vi "Is String Data Source Terminal Connected to Add States SubVI.vi"(7 "Wires Traversed in (for recursion)":refnum<vi>[](array[refnum]), 8 "error in (no error)":errorcluster, 11 "Wire":refnum<vi>) -> (0 "error out":errorcluster, 2 "Connected to Add States?":bool, 3 "Add States SubVI":refnum<vi>, 5 "Wires Traversed out":refnum<vi>[](array[refnum]))   [LabVIEW 2013, in "JKI State Machine API.lvlib"]
uses:
  JKI State Machine API.lvlib
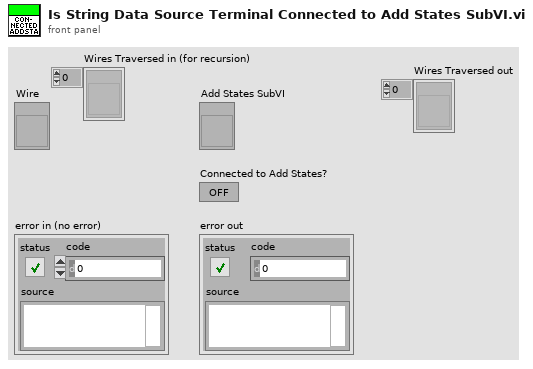
[diagram p1: front panel]
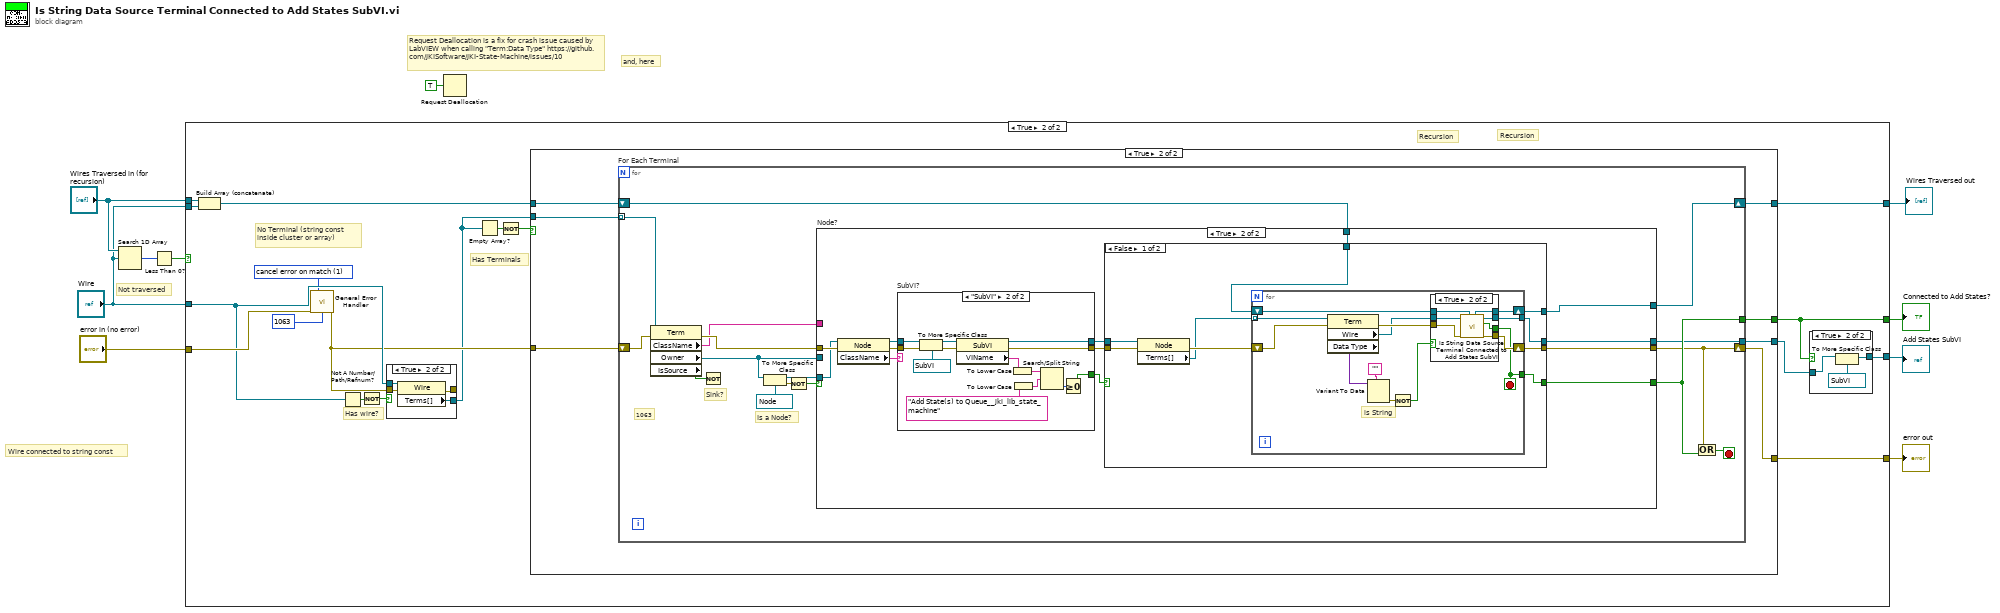
[diagram p0: block diagram]
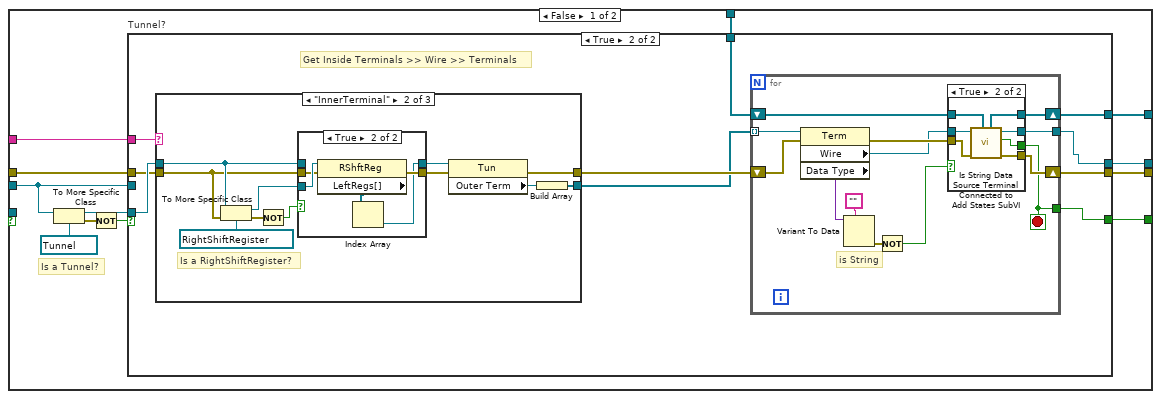
[diagram p5: hidden frame]
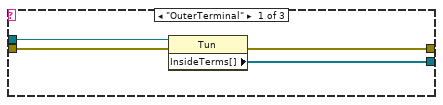
[diagram p7: hidden frame]
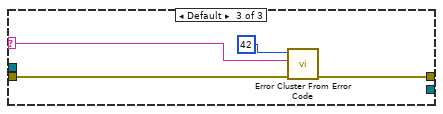
[diagram p9: hidden frame]
diagram:
  # "and, here"
  # "Request Deallocation is a fix for crash issue caused by LabVIEW when calling \"Term:Data Type\" https://github.com/JKISoftware/JKI-State-Machine/issues/10"
  # "Not traversed"
  # "Wire connected to string const"
  n1 = Search 1D Array(1D array="Wires Traversed in (for recursion)", element="Wire") -> (index of element=w6:i32)  [unwired: 1 in]
  n2 = Less Than 0?(x=w6) -> (x < 0?=w5:bool)
  n3 = case shown="True" w5 {
    tunnel: "error in (no error)" -> [w11 w30]
    tunnel: "Wire" -> [_ w29]
    tunnel: [w11 w21] -> w9
    tunnel: [_ w20] -> w8
    tunnel: [_ w18] -> w7
    tunnel: "Wires Traversed in (for recursion)" -> [w12 w16]
    tunnel: "Wire" -> [_ w15]
    tunnel: [w12 w13] -> w2
    frame False {
    }
    frame True {
      w22 = 1 items=["no exception", "cancel error on match", "set error on match"] ("[exception action] (none:0)")
      # "Recursion"
      # "Recursion"
      # "Has Terminals"
      # "Has wire?"
      # "No Terminal (string const inside cluster or array)"
      n4 = Build Array (concatenate)(w16, w15) -> (w14:refnum<vi>[])
      n5 = call <vilib>:"General Error Handler.vi"("error in (no error)"=w30, "[exception action] (none:0)"=w22, "[exception code]"=1063 ("[error code] (0)")) -> ("error out"=w23:errorcluster)  [unwired: 8 in, 4 out]
      n6 = Not A Number/Path/Refnum?(number/path/refnum=w29) -> (NaN/Path/Refnum?=w25:bool)
      n7 = Not(x=w25) -> (.not. x?=w26:bool)
      n8 = case shown="True" w26 {
        tunnel: w29 -> [_ w197]
        tunnel: [_ w196] -> w17
        tunnel: [w193 w194] -> _
        tunnel: w23 -> [w193 w195]
        frame False {
        }
        frame True {
          n9 = property class="Wire"(reference=w197, error in=w195) -> (error out=w194:errorcluster, "Terms[]"=w196:refnum<vi>[])  [unwired: 1 out]
        }
      }
      n10 = Empty Array?(array=w17) -> (empty?=w27:bool)
      n11 = Not(x=w27) -> (.not. x?=w28:bool)
      n12 = case shown="True" w28 {
        tunnel: [_ w41] -> w20
        tunnel: [_ w40] -> w21
        tunnel: w23 -> [_ w39]
        tunnel: w17 -> [_ w37]
        tunnel: [_ w38] -> w19
        tunnel: w14 -> [w34 w36]
        tunnel: [w34 w35] -> w13
        frame False {
        }
        frame True {
          n13 = for "For Each Terminal" {
            shift-right: [w52] -> w40
            shift-left: w39 -> [w56]
            tunnel: [w53] -> w41
            tunnel: [w51] -> w38
            tunnel: w37 -> [w50] mode=indexing
            shift-right: [w42] -> w35
            shift-left: w36 -> [w43]
            stop <- w49 stop-if-true
            # "Is a Node?"
            # "1063"
            # "Sink?"
            n14 = property class="Term"(reference=w50, error in=w56) -> (error out=w57:errorcluster, "ClassName"=w48:string, "Owner"=w55:refnum<vi>, "IsSource"=w54:bool)  [unwired: 1 out]
            n15 = Not(x=w54) -> ()  [unwired: 1 out]
            n16 = To More Specific Class(target class=refnum<vi> refnum ("Node Refnum"), reference=w55) -> (specific class reference=w44:refnum<vi>, error out=w46:errorcluster)  [unwired: 1 in]
            n17 = Not(x=w46) -> (.not. x?=w45:bool)
            n18 = case "Node?" shown="True" w45 {
              tunnel: w57 -> [w64 w139]
              tunnel: [w63 w137] -> w52
              tunnel: [w61 w134] -> w53
              tunnel: w44 -> [_ w138]
              tunnel: w55 -> [w66 _]
              tunnel: [w62 w133] -> w51
              tunnel: w48 -> [w60 _]
              tunnel: w43 -> [w59 w131]
              tunnel: [w58 w130] -> w42
              frame False {
                # "Is a Tunnel?"
                n19 = To More Specific Class(target class=refnum<vi> refnum ("Tun Refnum"), reference=w66) -> (specific class reference=w67:refnum<vi>, error out=w69:errorcluster)  [unwired: 1 in]
                n20 = Not(x=w69) -> (.not. x?=w65:bool)
                n21 = case "Tunnel?" shown="True" w65 {
                  tunnel: w67 -> [_ w81]
                  tunnel: w66 -> [_ _]
                  tunnel: w64 -> [w71 w80]
                  tunnel: [w71 w78] -> w63
                  tunnel: [_ w77] -> w62
                  tunnel: [_ w76] -> w61
                  tunnel: w60 -> [_ w75]
                  tunnel: w59 -> [w70 w73]
                  tunnel: [w70 w72] -> w58
                  frame False {
                  }
                  frame True {
                    # "Get Inside Terminals >> Wire >> Terminals"
                    n22 = case shown="\"InnerTerminal\"" w75 {
                      selector: w75 -> [_ _ w105]
                      tunnel: w81 -> [w85 w93 _]
                      tunnel: w80 -> [w84 w91 w107]
                      tunnel: [w83 w96 w106] -> w79
                      tunnel: [w82 w94 _] -> w74
                      frame "OuterTerminal" {
                        n23 = property class="Tun"(reference=w85, error in=w84) -> (error out=w83:errorcluster, "InsideTerms[]"=w82:refnum<vi>[])  [unwired: 1 out]
                      }
                      frame "InnerTerminal" {
                        # "Is a RightShiftRegister?"
                        n24 = To More Specific Class(target class=refnum<vi> refnum ("RShftReg Refnum"), reference=w93, error in=w91) -> (specific class reference=w86:refnum<vi>, error out=w89:errorcluster)
                        n25 = Not(x=w89) -> (.not. x?=w87:bool)
                        n26 = case shown="True" w87 {
                          tunnel: w86 -> [_ w103]
                          tunnel: w93 -> [w98 _]
                          tunnel: [w98 w99] -> w92
                          tunnel: w91 -> [w97 w101]
                          tunnel: [w97 w100] -> w90
                          frame False {
                          }
                          frame True {
                            n27 = property class="RShftReg"(reference=w103, error in=w101) -> (error out=w100:errorcluster, "LeftRegs[]"=w102:refnum<vi>[])  [unwired: 1 out]
                            n28 = Index Array(array=w102) -> (element=w99:refnum<vi>)  [unwired: 1 in]
                          }
                        }
                        n29 = property class="Tun"(reference=w92, error in=w90) -> (error out=w96:errorcluster, "Outer Term"=w95:refnum<vi>)  [unwired: 1 out]
                        n30 = Build Array(w95) -> (w94:refnum<vi>[])
                      }
                      frame Default {
                        n31 = call <vilib>:"Error Cluster From Error Code.vi"("error in (no error)"=w107, "error message (\"\")"=w105, "error code (0)"=42) -> ("error out"=w106:errorcluster)  [unwired: 6 in]
                      }
                    }
                    n32 = for {
                      tunnel: w74 -> [w120] mode=indexing
                      shift-right: [w117] -> w78
                      shift-left: w79 -> [w119]
                      tunnel: [w116] -> w77
                      tunnel: [w115] -> w76
                      shift-right: [w112] -> w72
                      shift-left: w73 -> [w113]
                      stop <- w115 stop-if-true
                      # "is String"
                      n33 = property class="Term"(reference=w120, error in=w119) -> (error out=w118:errorcluster, "Wire"=w114:refnum<vi>, "Data Type"=w109:variant)  [unwired: 1 out]
                      n34 = Variant To Data(type="" ("error in (no error)"), Variant=w109) -> (error out=w110:errorcluster)  [unwired: 1 in, 1 out]
                      n35 = Not(x=w110) -> (.not. x?=w108:bool)
                      n36 = case shown="True" w108 {
                        tunnel: w114 -> [_ w125]
                        tunnel: w118 -> [w122 w129]
                        tunnel: [w122 w128] -> w117
                        tunnel: [_ w127] -> w115
                        tunnel: [_ w126] -> w116
                        tunnel: w113 -> [w121 w124]
                        tunnel: [w121 w123] -> w112
                        frame False {
                        }
                        frame True {
                          n37 = call "Is String Data Source Terminal Connected to Add States SubVI.vi"("Wires Traversed in (for recursion)"=w124, "error in (no error)"=w129, "Wire"=w125) -> ("error out"=w128:errorcluster, "Connected to Add States?"=w127:bool, "Add States SubVI"=w126:refnum<vi>, "Wires Traversed out"=w123:refnum<vi>[])  [unwired: 5 in]
                        }
                      }
                    }
                  }
                }
              }
              frame True {
                n38 = property class="Node"(reference=w138, error in=w139) -> (reference out=w141:refnum<vi>, error out=w140:errorcluster, "ClassName"=w142:string)
                n39 = case "SubVI?" shown="\"SubVI\"" w142 {
                  tunnel: w141 -> [w178 w191]
                  tunnel: w140 -> [w179 w188]
                  tunnel: [_ w180] -> w135
                  tunnel: [w179 w185] -> w136
                  tunnel: [w178 w184] -> w132
                  frame Default {
                  }
                  frame "SubVI" {
                    n40 = To More Specific Class(target class=refnum<vi> refnum ("SubVI Refnum"), reference=w191, error in=w188) -> (specific class reference=w190:refnum<vi>, error out=w189:errorcluster)
                    n41 = property class="SubVI"(reference=w190, error in=w189) -> (reference out=w184:refnum<vi>, error out=w185:errorcluster, "VIName"=w187:string)
                    n42 = To Lower Case(string=w187) -> (all lower case string=w183:string)
                    n43 = To Lower Case(string="Add State(s) to Queue__jki_lib_state_machine" ("VI Name")) -> (all lower case string=w182:string)
                    n44 = Search/Split String(string=w183, search string/char (-)=w182) -> (offset of match=w181:i32)  [unwired: 1 in, 2 out]
                    n45 = Greater Or Equal To 0?(x=w181) -> (x >= 0?=w180:bool)
                  }
                }
                n46 = case shown="False" w135 {
                  selector: w135 -> [_ w177]
                  tunnel: [w151 w175] -> w137
                  tunnel: w136 -> [w149 w175]
                  tunnel: [w146 w177] -> w134
                  tunnel: [w147 w176] -> w133
                  tunnel: w132 -> [w150 w176]
                  tunnel: w131 -> [w144 w174]
                  tunnel: [w143 w174] -> w130
                  frame False {
                    n47 = property class="Node"(reference=w150, error in=w149) -> (error out=w148:errorcluster, "Terms[]"=w145:refnum<vi>[])  [unwired: 1 out]
                    n48 = for {
                      tunnel: w145 -> [w164] mode=indexing
                      shift-right: [w161] -> w151
                      shift-left: w148 -> [w163]
                      tunnel: [w160] -> w147
                      tunnel: [w159] -> w146
                      shift-right: [w156] -> w143
                      shift-left: w144 -> [w157]
                      stop <- w159 stop-if-true
                      # "is String"
                      n49 = property class="Term"(reference=w164, error in=w163) -> (error out=w162:errorcluster, "Wire"=w158:refnum<vi>, "Data Type"=w153:variant)  [unwired: 1 out]
                      n50 = Variant To Data(type="" ("error in (no error)"), Variant=w153) -> (error out=w154:errorcluster)  [unwired: 1 in, 1 out]
                      n51 = Not(x=w154) -> (.not. x?=w152:bool)
                      n52 = case shown="True" w152 {
                        tunnel: w158 -> [_ w173]
                        tunnel: w162 -> [w166 w172]
                        tunnel: [w166 w171] -> w161
                        tunnel: [_ w170] -> w159
                        tunnel: [_ w169] -> w160
                        tunnel: w157 -> [w165 w168]
                        tunnel: [w165 w167] -> w156
                        frame False {
                        }
                        frame True {
                          n53 = call "Is String Data Source Terminal Connected to Add States SubVI.vi"("Wires Traversed in (for recursion)"=w168, "error in (no error)"=w172, "Wire"=w173) -> ("error out"=w171:errorcluster, "Connected to Add States?"=w170:bool, "Add States SubVI"=w169:refnum<vi>, "Wires Traversed out"=w167:refnum<vi>[])  [unwired: 5 in]
                        }
                      }
                    }
                  }
                  frame True {
                  }
                }
              }
            }
            n54 = Compound Arithmetic op=OR(w52, w53) -> (w49:bool)
          }
        }
      }
      n55 = case shown="True" w20 {
        tunnel: w19 -> [_ w32]
        tunnel: [_ w31] -> w18
        frame False {
        }
        frame True {
          n56 = To More Specific Class(target class=refnum<vi> refnum ("SubVI Refnum"), reference=w32) -> (specific class reference=w31:refnum<vi>)  [unwired: 1 in, 1 out]
        }
      }
    }
  }
  "Add States SubVI" <- w7
  "Connected to Add States?" <- w8
  "error out" <- w9
  "Wires Traversed out" <- w2
  n57 = Request Deallocation(TRUE ("flag")) -> ()
